vi "Polybackwards.vi"(2 "Coefficients":dbl[](array[numeric]) format="%.2e", 3 "Y input":dbl format="%.2f") -> (0 "Iterartions":i32, 1 "X output":dbl format="%.3f")   [LabVIEW 2010]
panel:
  # "A                  B x              Cx^2             Dx^3"
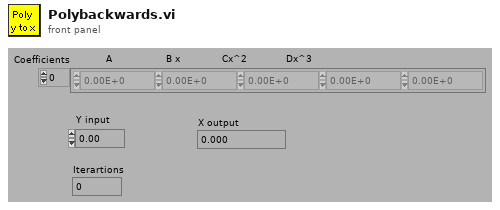
[diagram p1: front panel]
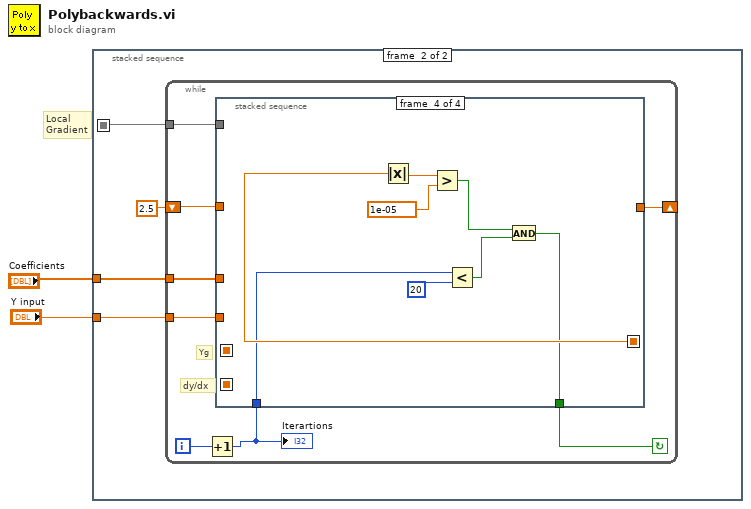
[diagram p0: block diagram]
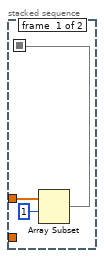
[diagram p2: hidden frame]
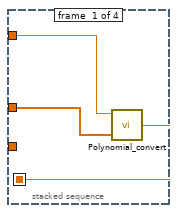
[diagram p3: hidden frame]
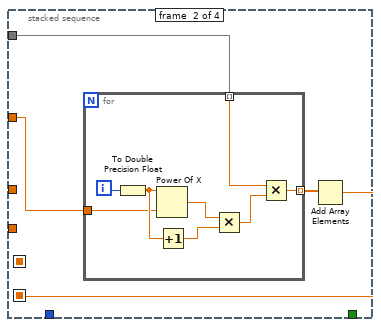
[diagram p4: hidden frame]
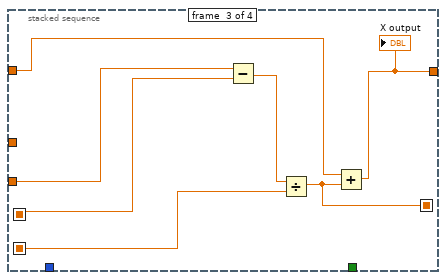
[diagram p5: hidden frame]
diagram:
  # "Local\nGradient"
  n1 = stacked-sequence {
    seq-local: [w3 _] -> [_ w7]
    tunnel: "Coefficients" -> [w5 w8]
    tunnel: "Y input" -> [_ w6]
    frame #0 {
      n2 = Array Subset(array=w5, index=1 ("Array Index")) -> (w3:dbl[])  [unwired: 1 in]
    }
    frame #1 {
      n3 = while {
        tunnel: w6 -> [w14]
        tunnel: w7 -> [w15]
        tunnel: w8 -> [w17]
        shift-left: 2.5 -> [w16]
        shift-right: [w13] -> _
        i -> [w11]
        stop <- w12 continue-if-true
        # "dy/dx"
        # "Yg"
        n4 = Increment(x=w11) -> (x+1=w10:i32)
        "Iterartions" <- w10
        n5 = stacked-sequence {
          seq-local: [w18 _ _ _] -> [_ _ w38 _]
          seq-local: [_ w21 _ _] -> [_ _ w36 _]
          seq-local: [_ _ w33 _] -> [_ _ _ w45]
          tunnel: w17 -> [w20 _ _ _]
          tunnel: w16 -> [w19 w24 w35 _]
          tunnel: w15 -> [_ w23 _ _]
          tunnel: w14 -> [_ _ w39 _]
          tunnel: [_ _ w34 _] -> w13
          tunnel: [_ _ _ w42] -> w12
          tunnel: w10 -> [_ _ _ w41]
          frame #0 {
            n6 = call "Polynomial_convert.vi"("Calib constants"=w20, "Voltage"=w19) -> ("Eng Values"=w18:dbl)  [unwired: 4 out]
          }
          frame #1 {
            n7 = for {
              tunnel: w24 -> [w28]
              tunnel: w23 -> [w26] mode=indexing
              tunnel: [w25] -> w22 mode=indexing
              i -> [w32]
              n8 = To Double Precision Float(number=w32) -> (double precision float=w29:dbl)
              n9 = Power Of X(1:w28, 2:w29) -> (0:w31:dbl)
              n10 = Increment(x=w29) -> (x+1=w30:dbl)
              n11 = Multiply(x=w31, y=w30) -> (x*y=w27:dbl)
              n12 = Multiply(x=w26, y=w27) -> (x*y=w25:dbl)
            }
            n13 = Add Array Elements(numeric array=w22) -> (sum=w21:dbl)
          }
          frame #2 {
            n14 = Subtract(x=w39, y=w38) -> (x-y=w37:dbl)
            n15 = Divide(x=w37, y=w36) -> (x/y=w33:dbl)
            n16 = Add(x=w35, y=w33) -> (x+y=w34:dbl)
            "X output" <- w34
          }
          frame #3 {
            n17 = Absolute Value(x=w45) -> (abs(x)=w47:dbl)
            n18 = Greater?(x=w47, y=1e-05) -> (0:w43:bool)
            n19 = Less?(x=w41, y=20 ("x")) -> (x < y?=w44:bool)
            n20 = And(x=w43, y=w44) -> (x .and. y?=w42:bool)
          }
        }
      }
    }
  }
